vi "Calculator.vi"() -> ()   [LabVIEW 2018]
panel:
  out "BoolText Indicator":string
  in  "stop":bool
  in  "plus":bool
  in  "^":bool
  in  ".":bool
  in  "=":bool
  in  "0":bool
  in  "minus":bool
  in  "tan":bool
  in  "2":bool
  in  "3":bool
  in  "1":bool
  in  "multiply":bool
  in  "cos":bool
  in  "5":bool
  in  "6":bool
  in  "4":bool
  in  "divide":bool
  in  "sin":bool
  in  "8":bool
  in  "9":bool
  in  "7":bool
  in  "AC":bool
  in  "Deg":bool
  in  "x!":bool
  in  "Rad":bool
  in  "%%":bool
  out "Display":string
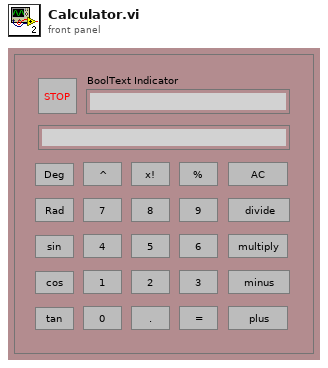
[diagram p1: front panel]
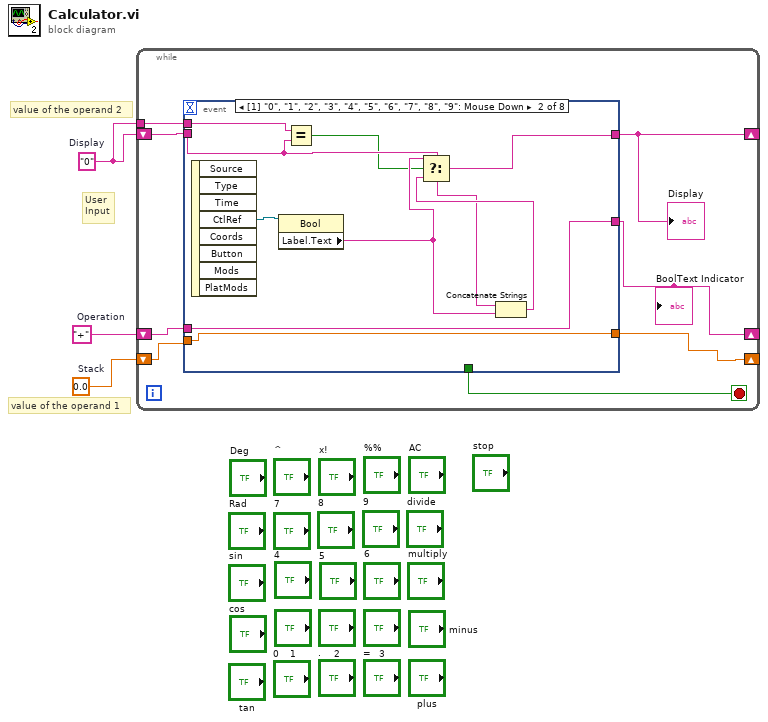
[diagram p0: block diagram]
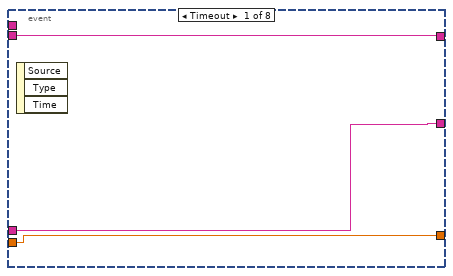
[diagram p2: hidden frame]
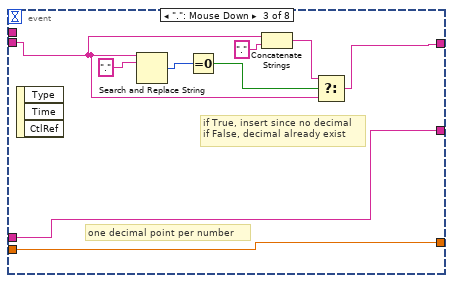
[diagram p3: hidden frame]
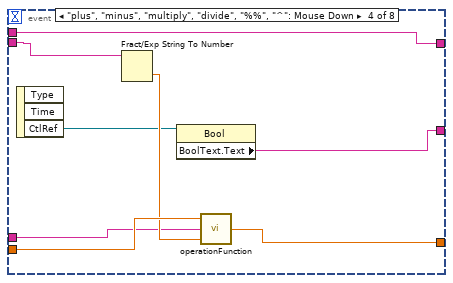
[diagram p4: hidden frame]
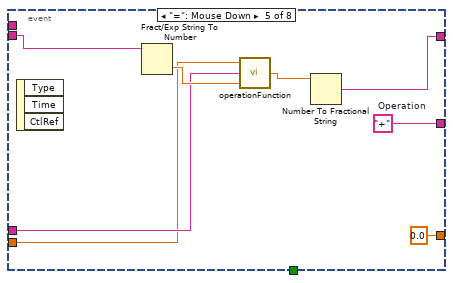
[diagram p5: hidden frame]
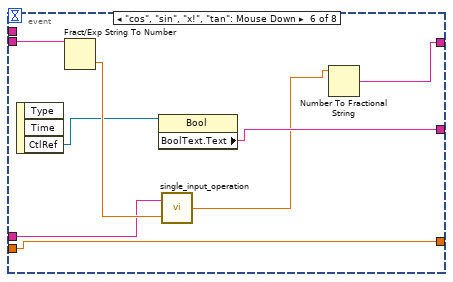
[diagram p6: hidden frame]
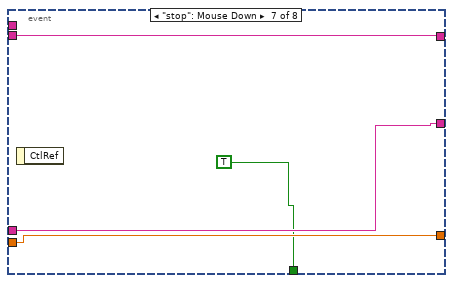
[diagram p7: hidden frame]
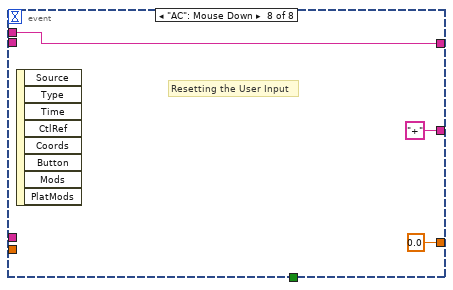
[diagram p8: hidden frame]
diagram:
  w1 = 0.0  # Stack
  w2 = "+"  # Operation
  w3 = "0"  # Display
  # "value of the operand 2"
  # "value of the operand 1"
  # "User\nInput"
  n1 = while {
    shift-right: [w9] -> _
    shift-left: w3 -> [w11]
    tunnel: w3 -> [w10]
    shift-right: [w5] -> _
    shift-left: w2 -> [w8]
    shift-right: [w6] -> _
    shift-left: w1 -> [w7]
    stop <- w4 stop-if-true
    n2 = event shown="[1] \"0\", \"1\", \"2\", \"3\", \"4\", \"5\", \"6\", \"7\", \"8\", \"9\": Mouse Down" {
      selector: _ -> [_ _ _ _ _ _ _ _]
      dyn-events: _ -> [_ _ _ _ _ _ _ _]
      timeout: _ -> [_ _ _ _ _ _ _ _]
      tunnel: [w14 w16 w25 w33 w42 w52 w60 "+" ("BoolText.Text")] -> w5
      tunnel: w11 -> [w12 w19 w28 w39 w48 w56 w58 _]
      tunnel: w10 -> [_ w18 _ w35 _ _ _ w63]
      tunnel: [w12 w21 w29 w35 w43 w49 w58 w63] -> w9
      tunnel: w8 -> [w14 w16 w25 w37 w46 w54 w60 _]
      tunnel: w7 -> [w13 w15 w24 w40 w45 w51 w59 _]
      tunnel: [w13 w15 w24 w36 0.0 ("Answer") w51 w59 0.0 ("Answer")] -> w6
      tunnel: [_ _ _ _ _ _ TRUE _] -> w4
      event Timeout {
        n3 = event-data() -> ()  [unwired: 1 in, 3 out]
      }
      event "0", "1", "2", "3", "4", "5", "6", "7", "8", "9": Mouse Down {
        n4 = event-data() -> ("CtlRef"=w20:refnum<vi>)  [unwired: 1 in, 7 out]
        n5 = property class="Bool"(reference=w20) -> ("Label.Text"=w23:string)  [unwired: 1 in, 2 out]
        n6 = Equal?(x=w18, y=w19) -> (x = y?=w17:bool)
        n7 = Concatenate Strings(w19, w23) -> (w22:string)
        n8 = Select(t=w23, s=w17, f=w22) -> (s? t:f=w21:string)
      }
      event ".": Mouse Down {
        # "if True, insert since no decimal\nif False, decimal already exist"
        # "one decimal point per number"
        n9 = event-data() -> ()  [unwired: 1 in, 3 out]
        n10 = Search and Replace String(input string=w28, search string=".") -> (number of replacements=w31:i32)  [unwired: 6 in, 3 out]
        n11 = Equal To 0?(x=w31) -> (x = 0?=w30:bool)
        n12 = Concatenate Strings(w28, "." ("search string")) -> (w26:string)
        n13 = Select(t=w26, s=w30, f=w28) -> (s? t:f=w29:string)
      }
      event "plus", "minus", "multiply", "divide", "%%", "^": Mouse Down {
        n14 = event-data() -> ("CtlRef"=w34:refnum<vi>)  [unwired: 1 in, 2 out]
        n15 = Fract/Exp String To Number(string=w39) -> (number=w38:dbl)  [unwired: 3 in, 1 out]
        n16 = property class="Bool"(reference=w34) -> ("BoolText.Text"=w33:string)  [unwired: 1 in, 2 out]
        n17 = call "operationFunction.vi"("y"=w38, "Operation"=w37, "x"=w40) -> ("Answer"=w36:dbl)
      }
      event "=": Mouse Down {
        w42 = "+"  # Operation
        n18 = event-data() -> ()  [unwired: 1 in, 3 out]
        n19 = Fract/Exp String To Number(string=w48) -> (number=w47:dbl)  [unwired: 3 in, 1 out]
        n20 = call "operationFunction.vi"("y"=w47, "Operation"=w46, "x"=w45) -> ("Answer"=w44:dbl)
        n21 = Number To Fractional String(number=w44) -> (F-format string=w43:string)  [unwired: 3 in]
      }
      event "cos", "sin", "x!", "tan": Mouse Down {
        n22 = event-data() -> ("CtlRef"=w53:refnum<vi>)  [unwired: 1 in, 2 out]
        n23 = Fract/Exp String To Number(string=w56) -> (number=w55:dbl)  [unwired: 3 in, 1 out]
        n24 = property class="Bool"(reference=w53) -> ("BoolText.Text"=w52:string)  [unwired: 1 in, 2 out]
        n25 = call "single_input_operation.vi"("Operand"=w55, "Operator"=w54) -> ("Result"=w50:dbl)
        n26 = Number To Fractional String(number=w50) -> (F-format string=w49:string)  [unwired: 3 in]
      }
      event "stop": Mouse Down {
        n27 = event-data() -> ()  [unwired: 1 in, 1 out]
      }
      event "AC": Mouse Down {
        # "Resetting the User Input"
        n28 = event-data() -> ()  [unwired: 1 in, 8 out]
      }
    }
    "Display" <- w9
    "BoolText Indicator" <- w5
  }
